vi "Move Relative.vi"(4 "error in (no error)":errorcluster, 5 "Position (0 units)":dbl format="%.6f", 6 "Axis (1)":i32=1 min=1 max=3, 7 "VISA resource name":refnum<visa-resource-name>) -> (0 "error out":errorcluster, 3 "VISA resource name out":refnum<visa-resource-name>)   [LabVIEW 2018, in "Newport ESP301.lvlib"]
doc: "This command initiates a relative motion. When received, the selected axis <B>Axis (1)</B> will move, with the predefined acceleration and velocity, to a relative position <B>Position (0 units)</B> units away from the current position. If the requested axis is member of a group, this command does not initiate the desired motion. Instead, error xx31, \"COMMAND NOT ALLOWED DUE TO GROUP ASSIGNMENT\" is generated. Refer HL and HC commands to move along a line or an arc.\nIf this command is issued when trajectory mode for this axis is not in trapezoidal or s-curve mode, the controller returns error xx32, “INVALID TRAJECTORY MODE FOR MOVING”.\n<B>NOTE:</B> Even though the command is accepted while a motion is in progress, care should\nbe taken not to reverse direction of motion."
uses:
  Newport ESP301.lvlib
panel:
  out "concatenated string":string
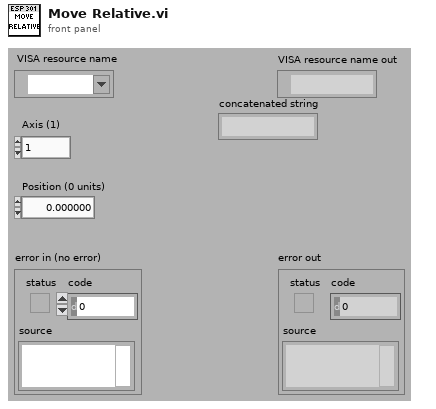
[diagram p1: front panel]
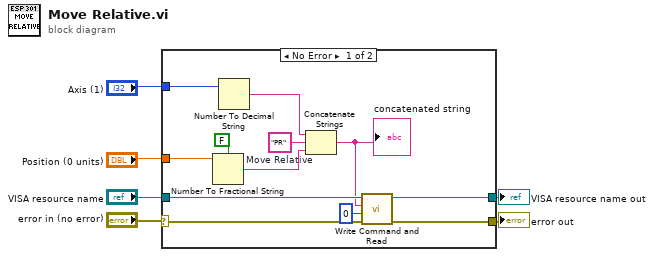
[diagram p0: block diagram]
diagram:
  n1 = case shown="No Error" "error in (no error)" {
    selector: "error in (no error)" -> [w15 w20]
    tunnel: [w17 w20] -> w6
    tunnel: "VISA resource name" -> [w18 w19]
    tunnel: [w16 w19] -> w5
    tunnel: "Axis (1)" -> [w10 _]
    tunnel: "Position (0 units)" -> [w9 _]
    frame No Error {
      w14 = "PR"  # Move Relative
      n2 = Number To Fractional String(use system decimal point (T)=FALSE ("utiliser le séparateur décimal du système (V)"), number=w9) -> (F-format string=w13:string)  [unwired: 2 in]
      n3 = Number To Decimal String(number=w10) -> (decimal integer string=w12:string)  [unwired: 1 in]
      n4 = Concatenate Strings(w12, w14, w13) -> (w11:string)
      "concatenated string" <- w11
      n5 = call "Write Command and Read.vi"("error in (no error)"=w15, "Bytes to read (100)"=u32 0, "Command"=w11, "VISA resource name"=w18) -> ("error out"=w17:errorcluster, "VISA resource name out"=w16:refnum<visa-resource-name>)  [unwired: 3 in, 1 out]
    }
    frame Error {
    }
  }
  "error out" <- w6
  "VISA resource name out" <- w5
